vi "RFSA 5668 Scanning Speed Benchmark Multi Record IQ.vi"() -> ()   [LabVIEW 2017]
doc: "Demonstrates the basics of I/Q acquisition using the RF vector signal analyzer. The example shows how to configure the <B>Clock Source</B>, <B>Reference Level</B>, <B>Carrier Frequency</B>, <B>I/Q rate</B>, <B>Samples per Record</B>, and I/Q acquisition type parameters. This example also reads and plots the I/Q data. The NI-RFSA multiple record acquisition does not acquire data continuously. There is a time gap between the end of each record and the beginning of the next acquisition."
uses:
  <vilib>/Utility/error.llb/DialogType.ctl
  <vilib>/Analysis/4window.llb/windowTd.ctl
  <vilib>/measure/maspectr.llb/FFT Power Spectrum and PSD for 1 Chan (CDB).vi
  <vilib>/measure/NI_MAPro.lvlib
  <vilib>/Analysis/NI_AALPro.lvlib
panel:
  out "size(s)":i32
  in  "Stop Carrier Frequency (Hz)":dbl=6000000000.0 format="%#_6p"
  in  "Resource Name 2":refnum<k15>="RFSG" caption="resource name"
  out "Waveform Graph 5":cluster{"f0":dbl, "df":dbl, "magnitude":dbl[]}(graph)
  out "Waveform Graph 4":cluster{"f0":dbl, "df":dbl, "magnitude":dbl[]}(graph)
  out "Waveform Graph 3":cluster{"f0":dbl, "df":dbl, "magnitude":dbl[]}(graph)
  out "Waveform Graph 2":cluster{"f0":dbl, "df":dbl, "magnitude":dbl[]}(graph)
  out "Waveform Graph":cluster{"f0":dbl, "df":dbl, "magnitude":dbl[]}(graph)
  in  "Start Carrier Frequency (Hz)":dbl=4000000000.0 format="%#_6p"
  in  "Resource Name":refnum<k15>="RFSA"
  in  "Reference Level (dBm)":dbl format="%.2f"
  # "External LO1 Generator"
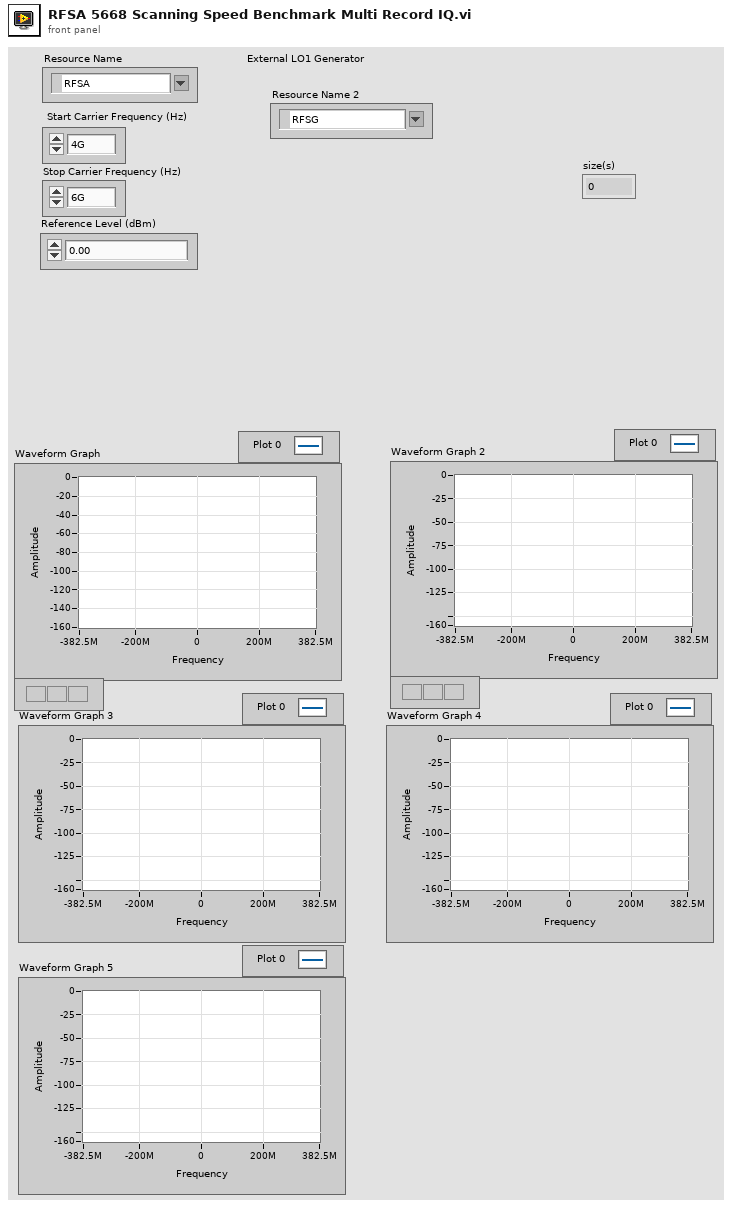
[diagram p1: front panel]
types:
  T1 = typedef "DialogType.ctl" = u16
  T2 = typedef "NI_AALPro.lvlib/windowTd.ctl" = u32
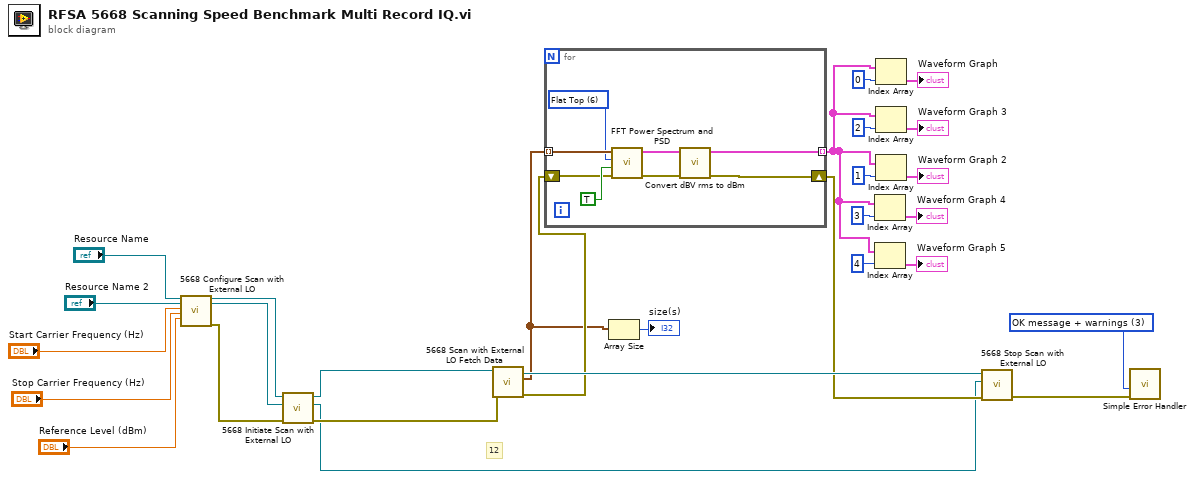
[diagram p0: block diagram]
diagram:
  w28 = T1 3 items=["no dialog", "OK message", "continue or stop message", "OK message + warnings", "continue/stop + warnings"] ("type of dialog (OK msg:1)")
  # "12"
  n1 = call "5668 Configure Scan with External LO.vi"("IVI Refnum in"="Resource Name", "Resource Name RFSG LO Generation"="Resource Name 2", "Start Carrier Frequency (Hz)"="Start Carrier Frequency (Hz)", "Stop Carrier Frequency (Hz)"="Stop Carrier Frequency (Hz)", "Reference Level (dBm)"="Reference Level (dBm)") -> ("RFSA Instrument Handle Out"=w25:refnum<k15>, "RFSG instrument handle out"=w3:refnum<k15>, "error out"=w8:errorcluster)  [unwired: 12 in]
  n2 = call "5668 Initiate Scan with External LO.vi"("error in (no error)"=w8, "RFSG instrument handle in"=w3, "RFSA Instrument Handle In"=w25) -> ("error out"=w10:errorcluster, "RFSG Instrument Handle Out"=w6:refnum<k15>, "RFSA Instrument Handle Out"=w9:refnum<k15>)  [unwired: 6 in]
  n3 = call "5668 Scan with External LO Fetch Data.vi"("error in (no error)"=w10, "RFSA Instrument Handle In"=w9) -> ("error out"=w19:errorcluster, "Data"=w2:waveform(cdb)[], "RFSA Instrument Handle Out"=w27:refnum<k15>)  [unwired: 7 in]
  n4 = for {
    tunnel: w2 -> [w36] mode=indexing
    tunnel: [w31] -> w17 mode=indexing
    shift-right: [w32] -> w18
    shift-left: w19 -> [w35]
    w30 = T2 6 items=["Rectangle"=0, "Hanning"=1, "Hamming"=2, "Blackman-Harris"=3, "Exact Blackman"=4, "Blackman"=5, "Flat Top"=6, "4 Term B-Harris "=7, "7 Term B-Harris"=8, "Low Sidelobe"=9, "Blackman Nuttall"=11, "Triangle"=30, "Bartlett-Hanning"=31, "Bohman"=32, "Parzen"=33, "Welch"=34, "Kaiser"=60, "Dolph-Chebyshev"=61, "Gaussian"=62] ("window")
    n5 = call-poly <vilib>:"FFT Power Spectrum and PSD.vi"("error in (no error)"=w35, "dB On (F)"=TRUE, "window"=w30, "time signal"=w36) -> ("error out"=w33:errorcluster, "Power Spectrum / PSD"=w34:cluster{"f0":dbl, "df":dbl, "magnitude":dbl[]})  [unwired: 4 in, 2 out]
    n6 = call "Convert dBV rms to dBm.vi"("error in (no error)"=w33, "Power Spectrum / PSD (dBV rms)"=w34) -> ("error out"=w32:errorcluster, "Power Spectrum / PSD (dBm)"=w31:cluster{"f0":dbl, "df":dbl, "magnitude":dbl[]})  [unwired: 8 in]
  }
  n7 = Array Size(array=w2) -> (size(s)=→"size(s)":i32)
  n8 = Index Array(array=w17, index=3) -> (element=→"Waveform Graph 4":cluster{"f0":dbl, "df":dbl, "magnitude":dbl[]})
  n9 = Index Array(array=w17, index=4) -> (element=→"Waveform Graph 5":cluster{"f0":dbl, "df":dbl, "magnitude":dbl[]})
  n10 = Index Array(array=w17, index=0) -> (element=→"Waveform Graph":cluster{"f0":dbl, "df":dbl, "magnitude":dbl[]})
  n11 = Index Array(array=w17, index=2) -> (element=→"Waveform Graph 3":cluster{"f0":dbl, "df":dbl, "magnitude":dbl[]})
  n12 = Index Array(array=w17, index=1) -> (element=→"Waveform Graph 2":cluster{"f0":dbl, "df":dbl, "magnitude":dbl[]})
  n13 = call "5668 Stop Scan with External LO.vi"("error in (no error)"=w18, "RFSG Instrument Handle In"=w6, "RFSA Instrument Handle In"=w27) -> ("error out"=w7:errorcluster)  [unwired: 8 in]
  n14 = call <vilib>:"Simple Error Handler.vi"("type of dialog (OK msg:1)"=w28, "error in (no error)"=w7) -> ()  [unwired: 3 in, 5 out]
